vi "Graph-Single.vi"() -> ()   [LabVIEW 2020]
panel:
  out "Graph-Array":dbl[](graph)
  out "Graph-Cluster":cluster{"x0":i32, "dx":i32, dbl[]}(graph)
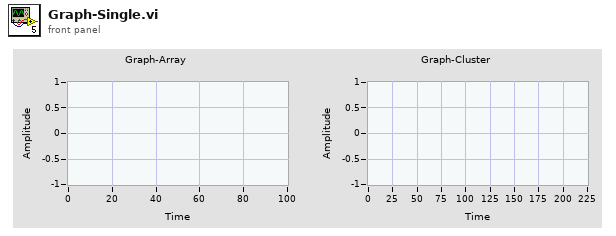
[diagram p1: front panel]
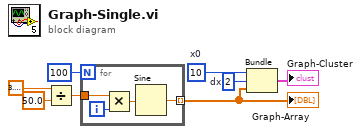
[diagram p0: block diagram]
diagram:
  w6 = 10  # x0
  w7 = 2  # dx
  n1 = Divide(x=3.141592653589793, y=50.0) -> (x/y=w1:dbl)
  n2 = for {
    N: 100 -> [_]
    tunnel: [w12] -> w4 mode=indexing
    tunnel: w1 -> [w9]
    i -> [w11]
    n3 = Multiply(x=w9, y=w11) -> (x*y=w10:dbl)
    n4 = Sine(x=w10) -> (sin(x)=w12:dbl)
  }
  "Graph-Array" <- w4
  n5 = Bundle("x0"=w6, "dx"=w7, w4) -> (→"Graph-Cluster":cluster{"x0":i32, "dx":i32, dbl[]})  [unwired: 1 in]
